vi "parse.vi"(8 "error in (no error)":errorcluster, 10 "DynamicFrameParser":refnum<class "DynamicFrameParser.lvclass">, 11 "FAILC in":refnum<class "FAILC.lvclass">) -> (0 "error out":errorcluster, 2 "ParseSuccessful":bool, 3 "FAILC out":refnum<class "FAILC.lvclass">)   [LabVIEW 2016, in "RTFAILC.lvlib" / "FAILC.lvclass"]
uses:
  FAILC.lvclass
  Common_RT_Modbus/DynamicFrameParser/DynamicFrameParser.lvclass
  Common_RT_ILC/ILC/ILC.lvclass
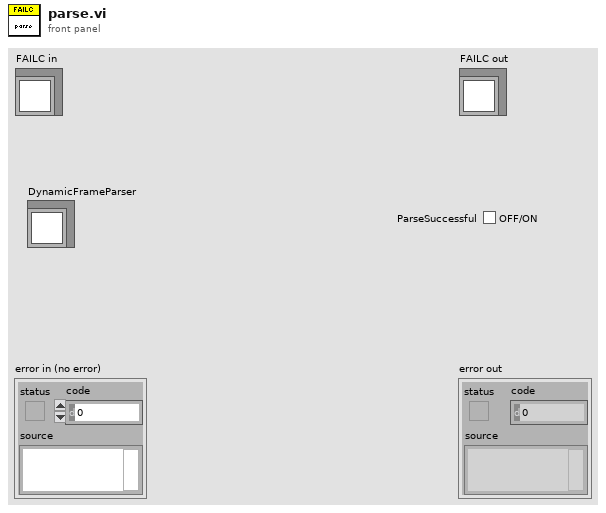
[diagram p1: front panel]
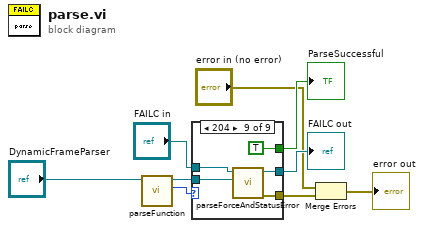
[diagram p0: block diagram]
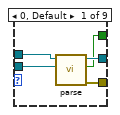
[diagram p2: hidden frame]
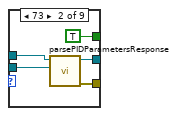
[diagram p3: hidden frame]
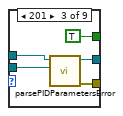
[diagram p4: hidden frame]
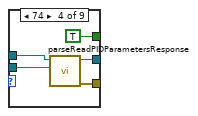
[diagram p5: hidden frame]
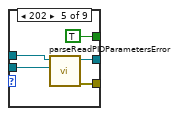
[diagram p6: hidden frame]
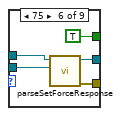
[diagram p7: hidden frame]
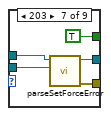
[diagram p8: hidden frame]
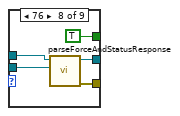
[diagram p9: hidden frame]
diagram:
  n1 = call "parseFunction.vi"("FrameParser in"="DynamicFrameParser") -> ("Function"=w8:u8, "FrameParser out"=w6:refnum<class "DynamicFrameParser.lvclass">)  [unwired: 8 in, 1 out]
  n2 = case shown="204" w8 {
    tunnel: "FAILC in" -> [w14 w19 w24 w29 w34 w39 w44 w49 w54]
    tunnel: w6 -> [w13 w18 w22 w26 w31 w38 w43 w48 w53]
    tunnel: [w12 w16 w23 w28 w33 w37 w42 w47 w52] -> w5
    tunnel: [w11 TRUE ("ParseSuccessful") TRUE ("ParseSuccessful") TRUE ("ParseSuccessful") TRUE ("ParseSuccessful") TRUE ("ParseSuccessful") TRUE ("ParseSuccessful") TRUE ("ParseSuccessful") TRUE ("ParseSuccessful")] -> w4
    tunnel: [w10 w17 w21 w27 w32 w36 w41 w46 w51] -> w3
    frame 0, Default {
      n3 = call-parent "parse.vi"("DynamicFrameParser"=w13, "ILC in"=w14) -> ("error out"=w10:errorcluster, "ParseSuccessful"=w11:bool, "ILC out"=w12:refnum<class "FAILC.lvclass">)  [unwired: 7 in]
    }
    frame 73 {
      n4 = call "parsePIDParametersResponse.vi"("DynamicFrameParser"=w18, "FAILC in"=w19) -> ("error out"=w17:errorcluster, "FAILC out"=w16:refnum<class "FAILC.lvclass">)  [unwired: 8 in]
    }
    frame 201 {
      n5 = call "parsePIDParametersError.vi"("DynamicFrameParser"=w22, "FAILC in"=w24) -> ("error out"=w21:errorcluster, "FAILC out"=w23:refnum<class "FAILC.lvclass">)  [unwired: 8 in]
    }
    frame 74 {
      n6 = call "parseReadPIDParametersResponse.vi"("DynamicFrameParser"=w26, "FAILC in"=w29) -> ("error out"=w27:errorcluster, "FAILC out"=w28:refnum<class "FAILC.lvclass">)  [unwired: 8 in]
    }
    frame 202 {
      n7 = call "parseReadPIDParametersError.vi"("DynamicFrameParser"=w31, "FAILC in"=w34) -> ("error out"=w32:errorcluster, "FAILC out"=w33:refnum<class "FAILC.lvclass">)  [unwired: 8 in]
    }
    frame 75 {
      n8 = call-dynamic "parseSetForceResponse.vi"("DynamicFrameParser"=w38, "FAILC in"=w39) -> ("error out"=w36:errorcluster, "FAILC out"=w37:refnum<class "FAILC.lvclass">)  [unwired: 8 in]
    }
    frame 203 {
      n9 = call "parseSetForceError.vi"("DynamicFrameParser"=w43, "FAILC in"=w44) -> ("error out"=w41:errorcluster, "FAILC out"=w42:refnum<class "FAILC.lvclass">)  [unwired: 8 in]
    }
    frame 76 {
      n10 = call-dynamic "parseForceAndStatusResponse.vi"("DynamicFrameParser"=w48, "FAILC in"=w49) -> ("error out"=w46:errorcluster, "FAILC out"=w47:refnum<class "FAILC.lvclass">)  [unwired: 8 in]
    }
    frame 204 {
      n11 = call "parseForceAndStatusError.vi"("DynamicFrameParser"=w53, "FAILC in"=w54) -> ("error out"=w51:errorcluster, "FAILC out"=w52:refnum<class "FAILC.lvclass">)  [unwired: 8 in]
    }
  }
  "FAILC out" <- w5
  "ParseSuccessful" <- w4
  n12 = Merge Errors("error in (no error)", w3) -> (→"error out":errorcluster)
